vi "Resolve Value.vi"(4 "Value Name":string, 6 "Namespace":string, 7 "Folder":path, 8 "error in (no error)":errorcluster, 9 "Locals":map{string, string}(c390), 11 "BasicTemplater in":refnum<class "BasicTemplater.lvclass">) -> (0 "error out":errorcluster, 2 "Value":string, 3 "BasicTemplater out":refnum<class "BasicTemplater.lvclass">)   [LabVIEW 2020, in "HTTP Server.lvlib" / "BasicTemplater.lvclass"]
uses:
  BasicTemplater.lvclass
  C:/dev/lv20CE/relink/lv-http-server/HTTP Server/TemplateService/TemplateService.lvclass
  BasicTemplater.lvclass/BasicTemplater.ctl
  TemplateService/TemplateService.lvclass
  TemplateVariableResolver/TemplateValueResolver.lvclass
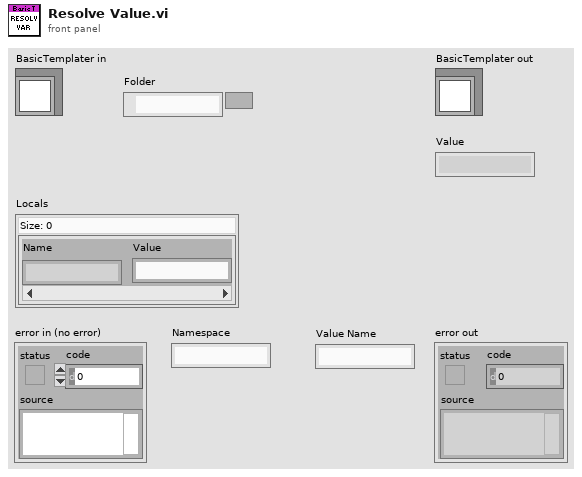
[diagram p1: front panel]
types:
  T1 = map{string, refnum<class "TemplateValueResolver.lvclass">}
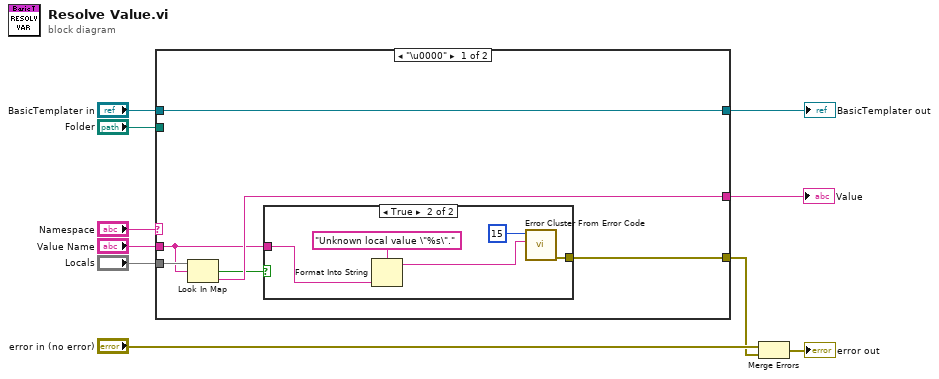
[diagram p0: block diagram]
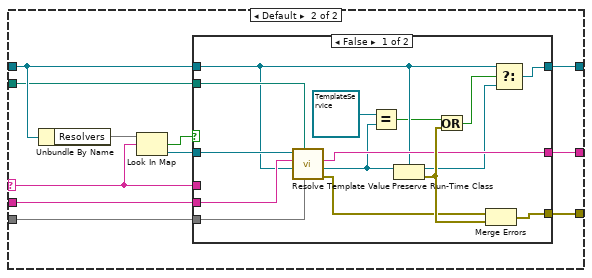
[diagram p3: hidden frame]
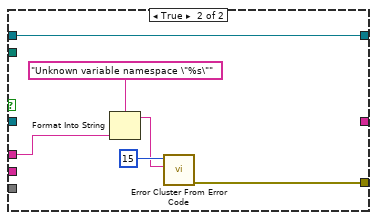
[diagram p4: hidden frame]
diagram:
  n1 = case shown="\"\"" "Namespace" {
    selector: "Namespace" -> [_ w31]
    tunnel: "Value Name" -> [w12 w30]
    tunnel: [w15 w29] -> w7
    tunnel: [w11 w28] -> w5
    tunnel: "BasicTemplater in" -> [w14 w25]
    tunnel: [w14 w24] -> w3
    tunnel: "Folder" -> [_ w23]
    tunnel: "Locals" -> [w16 w22]
    frame "\u0000" {
      n2 = Look In Map(map=w16, key=w12) -> (key not found?=w13:bool, value=w15:string)  [unwired: 1 in]
      n3 = case shown="True" w13 {
        tunnel: w12 -> [_ w19]
        tunnel: [_ w18] -> w11
        frame False {
        }
        frame True {
          n4 = Format Into String(format string="Unknown local value \"%s\".", w19) -> (resulting string=w17:string)  [unwired: 2 in, 1 out]
          n5 = call <vilib>:"Error Cluster From Error Code.vi"("error message (\"\")"=w17, "error code (0)"=15) -> ("error out"=w18:errorcluster)  [unwired: 7 in]
        }
      }
    }
    frame Default {
      n6 = Unbundle By Name(w25) -> ("Resolvers"=w32:T1)
      n7 = Look In Map(map=w32, key=w31) -> (key not found?=w27:bool, value=w26:refnum<class "TemplateValueResolver.lvclass">)  [unwired: 1 in]
      n8 = case shown="False" w27 {
        tunnel: w26 -> [w45 _]
        tunnel: w31 -> [_ w50]
        tunnel: w30 -> [w44 _]
        tunnel: [w43 _] -> w29
        tunnel: [w38 w53] -> w28
        tunnel: w25 -> [w41 w48]
        tunnel: [w39 w48] -> w24
        tunnel: w23 -> [w42 _]
        tunnel: w22 -> [w33 _]
        frame False {
          n9 = call-dynamic "Resolve Template Value.vi"("Locals"=w33, "Folder"=w42, "Template Service in"=w41, "Value Name"=w44, "TemplateVariableResolver in"=w45) -> ("error out"=w46:errorcluster, "Template Service"=w37:refnum<class "TemplateService.lvclass">, "Value"=w43:string)  [unwired: 4 in]
          n10 = Equal?(x=refnum<class "TemplateService.lvclass"> refnum, y=w37) -> (x = y?=w35:bool)
          n11 = Preserve Run-Time Class(object in=w37, 2:w41) -> (object out=w40:refnum<class "BasicTemplater.lvclass">, error out=w47:errorcluster)  [unwired: 1 in]
          n12 = Or(x=w35, y=w47) -> (x .or. y?=w34:bool)
          n13 = Merge Errors(w46, w47) -> (w38:errorcluster)
          n14 = Select(t=w41, s=w34, f=w40) -> (s? t:f=w39:refnum<class "BasicTemplater.lvclass">)
        }
        frame True {
          n15 = Format Into String(format string="Unknown variable namespace \"%s\"", w50) -> (resulting string=w49:string)  [unwired: 2 in, 1 out]
          n16 = call <vilib>:"Error Cluster From Error Code.vi"("error message (\"\")"=w49, "error code (0)"=15) -> ("error out"=w53:errorcluster)  [unwired: 7 in]
        }
      }
    }
  }
  "BasicTemplater out" <- w3
  "Value" <- w7
  n17 = Merge Errors("error in (no error)", w5) -> (→"error out":errorcluster)
